vi "DS11202Z MEAS.vi"(9 "参数":T1(array[ring]), 10 "通道":enum16{"Channel_1", "Channel_2"}(ring), 11 "TestIndex":i32) -> (0 "错误输出":errorcluster, 3 "ValueArry":dbl[](array[numeric]) format="%#_6f")   [LabVIEW 2015]
panel:
  out "读取缓冲区":string
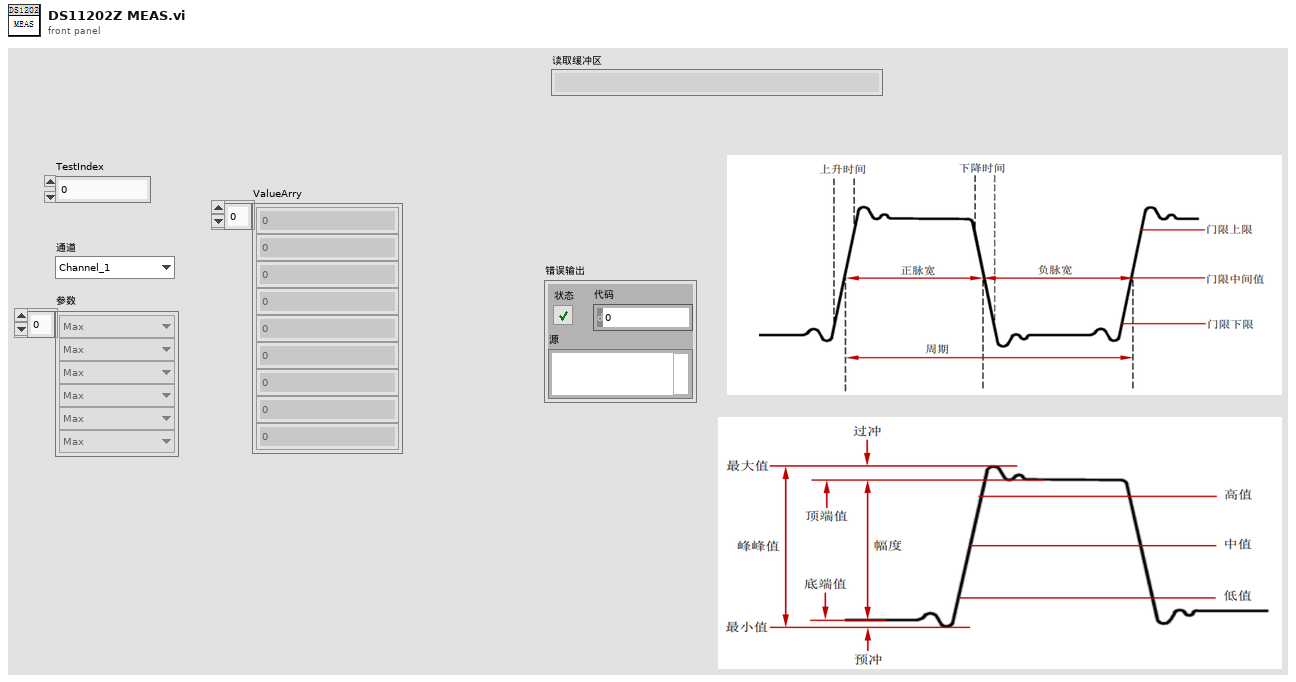
[diagram p1: front panel]
types:
  T1 = enum16{"Max", "Min", "Vpp", "Top", "Amp", "Avg", "Vrms", "Freq", "+Duty", "-Duty"}[]
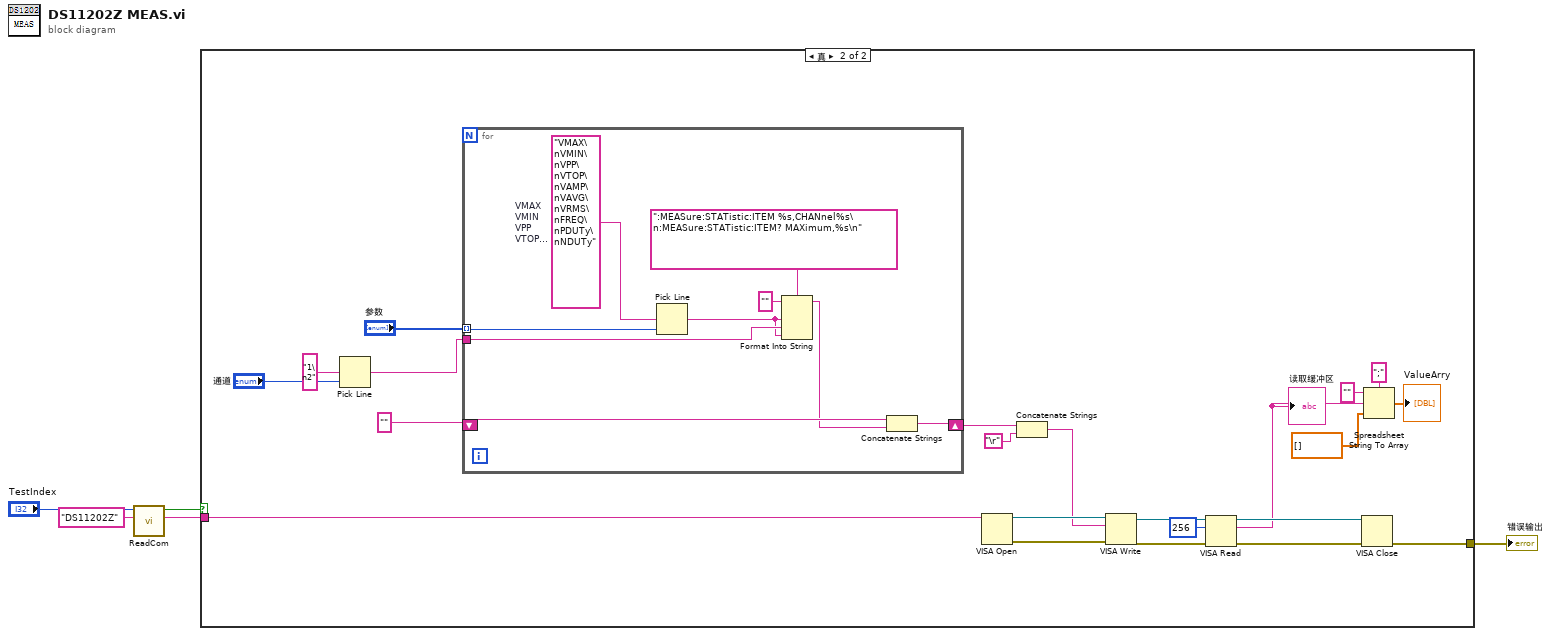
[diagram p0: block diagram]
diagram:
  n1 = call "ReadCom.vi"("仪器名称"="DS11202Z", "MyIndex"="TestIndex") -> ("COM"=w2:string, "OK?"=w1:bool)  [unwired: 7 in, 1 out]
  n2 = case shown="真" w1 {
    tunnel: [_ w18] -> w5
    tunnel: w2 -> [_ w6]
    frame False {
    }
    frame True {
      n3 = Pick Line(multi-line string="1\n2", line index="通道") -> (output string=w24:string)  [unwired: 1 in]
      n4 = for {
        tunnel: "参数" -> [w35] mode=indexing
        tunnel: w24 -> [w32]
        shift-right: [w31] -> w22
        shift-left: "" -> [w30]
        w36 = "VMAX\nVMIN\nVPP\nVTOP\nVAMP\nVAVG\nVRMS\nFREQ\nPDUTy\nNDUTy"  # VMAX VMIN VPP VTOP VAMP VAVG VRMS FREQ PDUTy NDUTy
        n5 = Pick Line(multi-line string=w36, line index=w35) -> (output string=w28:string)  [unwired: 1 in]
        n6 = Format Into String(format string=":MEASure:STATistic:ITEM %s,CHANnel%s\n:MEASure:STATistic:ITEM? MAXimum,%s\n" ("字符串"), initial string="" ("初始字符串"), w28, w32, w28) -> (resulting string=w29:string)  [unwired: 1 in, 1 out]
        n7 = Concatenate Strings(w30, w29) -> (w31:string)
      }
      n8 = VISA Open(VISA resource name=w6) -> (VISA resource name=w20:refnum<visa-resource-name>, error out=w19:errorcluster)  [unwired: 1 in, 3 out]
      n9 = Concatenate Strings(w22, "\r") -> (w12:string)
      n10 = VISA Write(VISA resource name=w20, write buffer=w12, error in (no error)=w19) -> (VISA resource name out=w15:refnum<visa-resource-name>, error out=w17:errorcluster)  [unwired: 1 out]
      n11 = VISA Read(VISA resource name=w15, byte count=u32 256 ("字节总数"), error in (no error)=w17) -> (VISA resource name out=w14:refnum<visa-resource-name>, read buffer=w11:string, error out=w16:errorcluster)  [unwired: 1 out]
      "读取缓冲区" <- w11
      n12 = VISA Close(VISA resource name=w14, error in (no error)=w16) -> (error out=w18:errorcluster)
      n13 = Spreadsheet String To Array(delimiter (Tab)=";" ("分隔符(Tab)"), format string="" ("格式字符串"), spreadsheet string=w11, array type (2D Dbl)=dbl[] []) -> (array=→"ValueArry":dbl[])
    }
  }
  "错误输出" <- w5
